vi "Simple Local State Callback.vi"(7 "Owner":refnum<class>, 8 "error in (no error)":errorcluster, 10 "Connection State":T1, 11 "Connection":refnum<class "Connection.lvclass">) -> (0 "error out":errorcluster)   [LabVIEW 2020]
uses:
  lv-stream/stream/Connection/Connection.lvclass
  lv-stream/stream/Connection State.ctl
  4439bedd-953a-4445-bdb5-6aaf4e7aeb87.vi
  lv-stream/stream/Stream/Stream.lvclass
  lv-stream/stream/Stream.lvlib
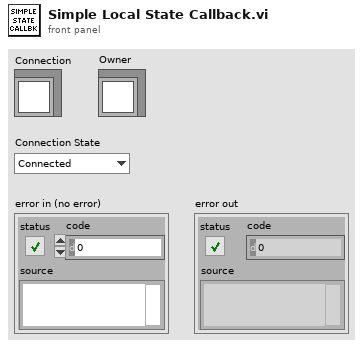
[diagram p1: front panel]
types:
  T1 = typedef "Stream.lvlib/Connection State.ctl" = enum16{"Connected", "Disconnected"}
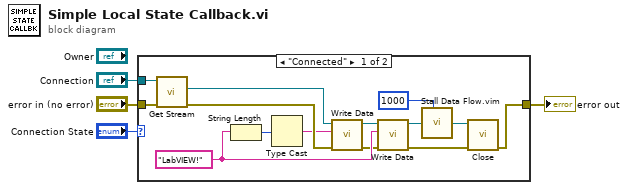
[diagram p0: block diagram]
diagram:
  n1 = case shown="\"Connected\"" "Connection State" {
    tunnel: "error in (no error)" -> [w17 w19]
    tunnel: "Connection" -> [w16 _]
    tunnel: [w5 w19] -> w1
    frame "Connected" {
      w11 = "LabVIEW!"
      n2 = call-dynamic "Get Stream.vi"("error in (no error)"=w17, "Connection in"=w16) -> ("error out"=w18:errorcluster, "Stream"=w15:refnum<class "Stream.lvclass">)  [unwired: 7 in, 1 out]
      n3 = String Length(string=w11) -> (length=w12:i32)
      n4 = Type Cast(x=w12) -> (*(type *) &x=w14:string)  [unwired: 1 in]
      n5 = call-dynamic "Write Data.vi"("error in (no error)"=w18, "Data"=w14, "Stream in"=w15) -> ("error out"=w7:errorcluster, "Stream out"=w13:refnum<class "Stream.lvclass">)  [unwired: 7 in]
      n6 = call-dynamic "Write Data.vi"("error in (no error)"=w7, "Data"=w11, "Stream in"=w13) -> ("error out"=w6:errorcluster, "Stream out"=w10:refnum<class "Stream.lvclass">)  [unwired: 7 in]
      n7 = call "Stall Data Flow.vim"("value in"=w10, "milliseconds to wait"=u32 1000) -> ("value out"=w8:refnum<class "Stream.lvclass">)  [unwired: 1 out]
      n8 = call-dynamic "Close.vi"("error in (no error)"=w6, "Stream in"=w8) -> ("error out"=w5:errorcluster)  [unwired: 8 in, 1 out]
    }
    frame "Disconnected" {
    }
  }
  "error out" <- w1
